vi "Ramp acceleration.vi"(9 "Numeric":dbl) -> (1 "Numeric 2":dbl)   [LabVIEW 2014]
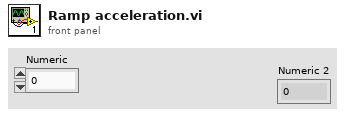
[diagram p1: front panel]
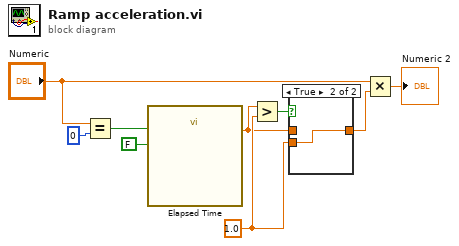
[diagram p0: block diagram]
diagram:
  w2 = 1.0
  n1 = Equal?(x="Numeric", y=0) -> (x = y?=w5:bool)
  n2 = call "Elapsed Time"("Reset"=w5, "Auto Reset"=FALSE ("Reset")) -> ("Elapsed Time (s)"=w1:dbl)  [unwired: 10 in, 7 out]
  n3 = Greater?(x=w1, y=w2) -> (0:w4:bool)
  n4 = case shown="True" w4 {
    tunnel: [w10 w11] -> w3
    tunnel: w2 -> [_ w11]
    tunnel: w1 -> [w10 _]
    frame False {
    }
    frame True {
    }
  }
  n5 = Multiply(x="Numeric", y=w3) -> (x*y=→"Numeric 2":dbl)
